vi "test_advanced_Doppler.vi"() -> ()   [LabVIEW 2009]
doc: "Copyright (C) 2009, Stepan A. Baranov\nweb: http://www.OCTLab.org/\nemail: stepan@baranov.su"
uses:
  OCTLib.dll
panel:
  out "version":string
  out "name":string
  out "error out":errorcluster
  out "window width radius":i32
  out "window height radius":i32
  out "width":i32
  out "height":i32
  in  "Small/Big":bool
  out "loop #":i32
  out "RSM_STAT time":u32
  out "LabView time":u32
  out "RSM_STAT Array":dbl[][](array[numeric])
  out "LabView Array":dbl[][](array[numeric])
  in  "stop":bool
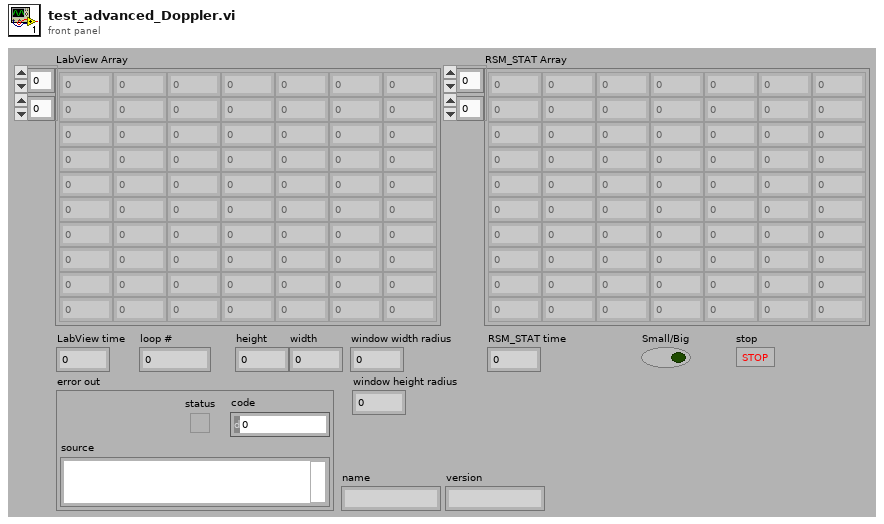
[diagram p1: front panel]
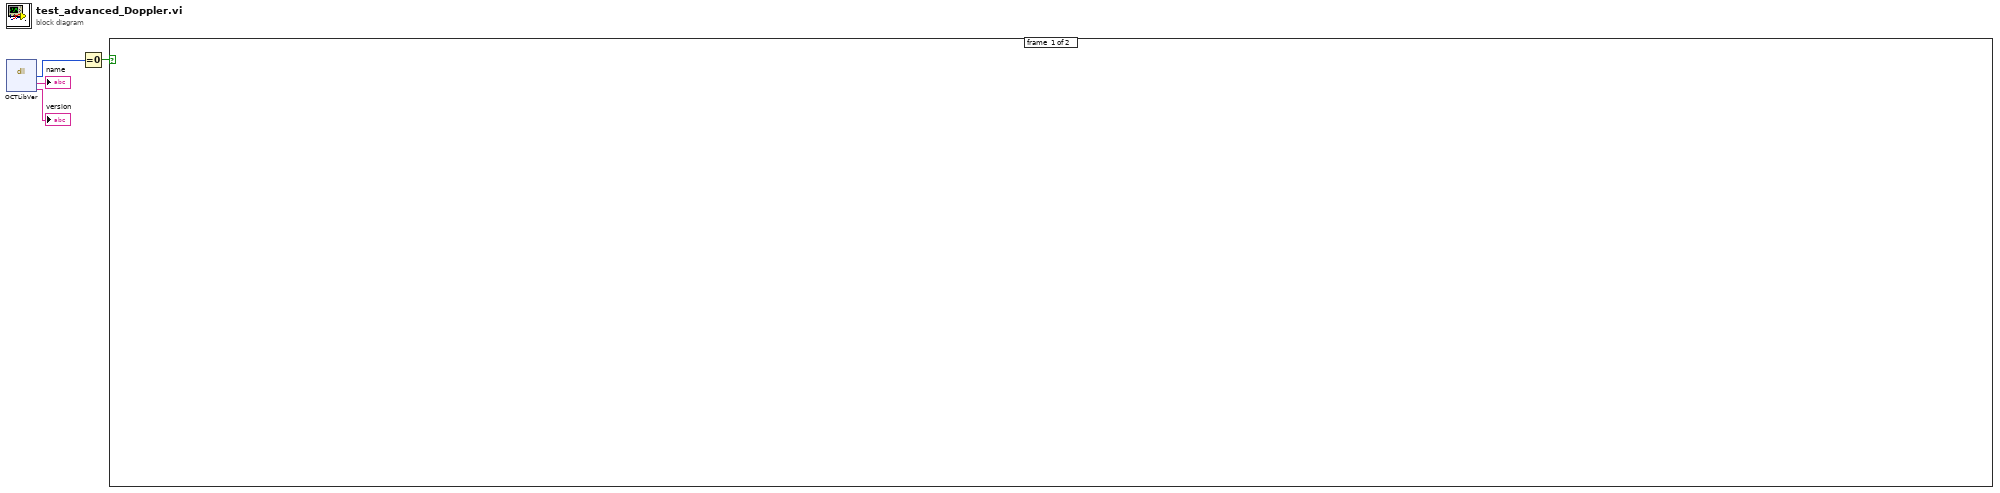
[diagram p0: block diagram]
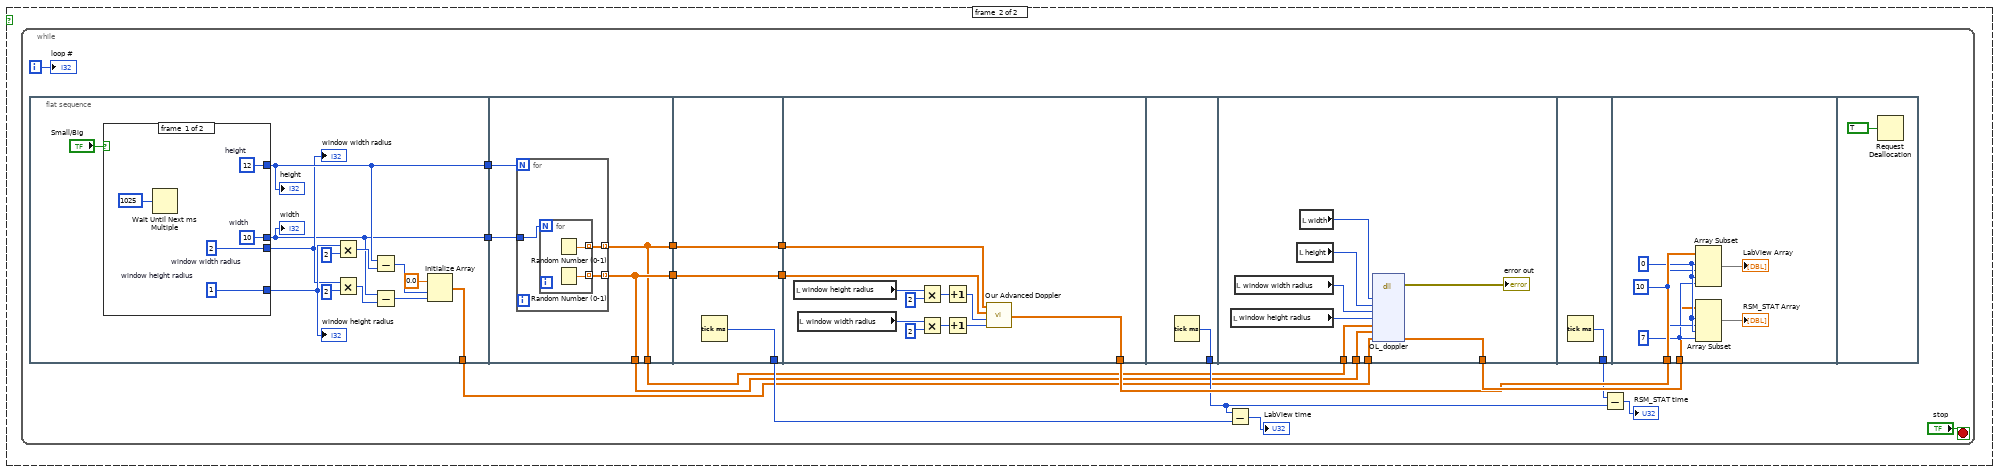
[diagram p2: hidden frame]
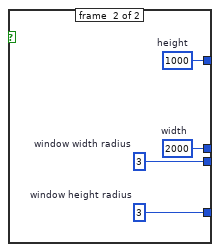
[diagram p3: hidden frame]
diagram:
  n1 = dll-call lib="OCTLib.dll" fn="OCTLibVer"() -> ("status"=w4:i8, "name"=→"name":string, "version"=→"version":string)  [unwired: 5 in, 2 out]
  n2 = Equal To 0?(x=w4) -> (x = 0?=w3:bool)
  n3 = case shown="True" w3 {
    frame #0 {
    }
    frame #1 {
      n4 = while {
        i -> [w14]
        stop <- "stop" stop-if-true
        n5 = flat-sequence {
          tunnel: [w25] -> w10
          tunnel: [w32] -> w9
          tunnel: [w23] -> w5
          tunnel: [w46] -> w13
          tunnel: [w46] -> w11
          tunnel: w10 -> [w48]
          tunnel: w9 -> [w47]
          tunnel: [w45] -> w8
          tunnel: [w45] -> w6
          tunnel: [w56] -> w19
          tunnel: [w55] -> w12
          tunnel: w11 -> [w55]
          tunnel: w8 -> [w54]
          tunnel: [w54] -> w7
          tunnel: [w57] -> w20
          tunnel: w12 -> [w66]
          tunnel: w7 -> [w67]
          tunnel: [w68] -> w16
          tunnel: w13 -> [w74]
          tunnel: [w77] -> w21
          tunnel: w6 -> [w73]
          tunnel: w5 -> [w70]
          tunnel: [w78] -> w17
          tunnel: w21 -> [w79]
          tunnel: w20 -> [w85]
          frame #0 {
            n6 = case shown="False" "Small/Big" {
              tunnel: [w39 w44] -> w32
              tunnel: [w40 w43] -> w25
              tunnel: [w37 w42] -> w34
              tunnel: [w36 w41] -> w26
              frame #0 {
                w36 = 2  # window width radius
                w37 = 1  # window height radius
                w40 = 10  # width
                w39 = 12  # height
                n7 = Wait Until Next ms Multiple(millisecond multiple=u32 1025) -> ()  [unwired: 1 out]
              }
              frame #1 {
                w41 = 3  # window width radius
                w42 = 3  # window height radius
                w43 = 2000  # width
                w44 = 1000  # height
              }
            }
            "height" <- w32
            "width" <- w25
            "window height radius" <- w34
            "window width radius" <- w26
            n8 = Multiply(x=w34, y=2) -> (x*y=w31:i32)
            n9 = Multiply(x=w26, y=2) -> (x*y=w27:i32)
            n10 = Subtract(x=w32, y=w31) -> (x-y=w30:i32)
            n11 = Subtract(x=w25, y=w27) -> (x-y=w24:i32)
            n12 = Initialize Array(0.0 ("element"), w30, w24) -> (w23:dbl[][])
          }
          frame #1 {
            n13 = for {
              N: w47 -> [_]
              tunnel: w48 -> [w51]
              tunnel: [w50] -> w46 mode=indexing
              tunnel: [w49] -> w45 mode=indexing
              n14 = for {
                N: w51 -> [_]
                tunnel: [w53] -> w50 mode=indexing
                tunnel: [w52] -> w49 mode=indexing
                n15 = Random Number (0-1)() -> (number: 0 to 1=w52:dbl)
                n16 = Random Number (0-1)() -> (number: 0 to 1=w53:dbl)
              }
            }
          }
          frame #2 {
            n17 = Tick Count (ms)() -> (millisecond timer value=w56:u32)
          }
          frame #3 {
            n18 = local read "window height radius"() -> (w65:i32)
            n19 = local read "window width radius"() -> (w60:i32)
            n20 = Multiply(x=w65, y=2) -> (x*y=w63:i32)
            n21 = Multiply(x=w60, y=2) -> (x*y=w61:i32)
            n22 = Increment(x=w63) -> (x+1=w58:i32)
            n23 = Increment(x=w61) -> (x+1=w59:i32)
            n24 = call "Our Advanced Doppler.vi"("Horizontal Window"=w59, "Vertical Window"=w58, "Imaginary Part"=w66, "Real Part"=w67) -> ("2D Doppler Image"=w57:dbl[][])
          }
          frame #4 {
            n25 = Tick Count (ms)() -> (millisecond timer value=w68:u32)
          }
          frame #5 {
            n26 = local read "window height radius"() -> (w71:i32)
            n27 = local read "window width radius"() -> (w72:i32)
            n28 = local read "height"() -> (w75:i32)
            n29 = local read "width"() -> (w76:i32)
            n30 = dll-call lib="OCTLib.dll" fn="OL_doppler"("width"=w76, "height"=w75, "window width radius"=w72, "window height radius"=w71, "Re"=w73, "Im"=w74, "data"=w70) -> (error out=→"error out":errorcluster, "data"=w77:dbl[][])  [unwired: 10 in, 1 out]
          }
          frame #6 {
            n31 = Tick Count (ms)() -> (millisecond timer value=w78:u32)
          }
          frame #7 {
            w82 = 10 ("length")
            w81 = 7 ("length")
            w83 = 0 ("index")
            n32 = Array Subset(array=w85, index (row)=w83, length (row)=w82, index (col)=w83, length (col)=w81) -> (→"LabView Array":dbl[][])
            n33 = Array Subset(array=w79, index (row)=w83, length (row)=w82, index (col)=w83, length (col)=w81) -> (→"RSM_STAT Array":dbl[][])
          }
          frame #8 {
            n34 = Request Deallocation(TRUE ("flag")) -> ()
          }
        }
        n35 = Subtract(x=w16, y=w19) -> (x-y=→"LabView time":u32)
        n36 = Subtract(x=w17, y=w16) -> (x-y=→"RSM_STAT time":u32)
        "loop #" <- w14
      }
    }
  }
